vi "图像DCT变换.vi"(11 "图像簇":T1) -> (3 "DCT变换结果":dbl[][][](array[numeric]))   [LabVIEW 2018]
uses:
  <vilib>/Analysis/2dsp.llb/2D DCT.vi
  <vilib>/Analysis/NI_AALPro.lvlib
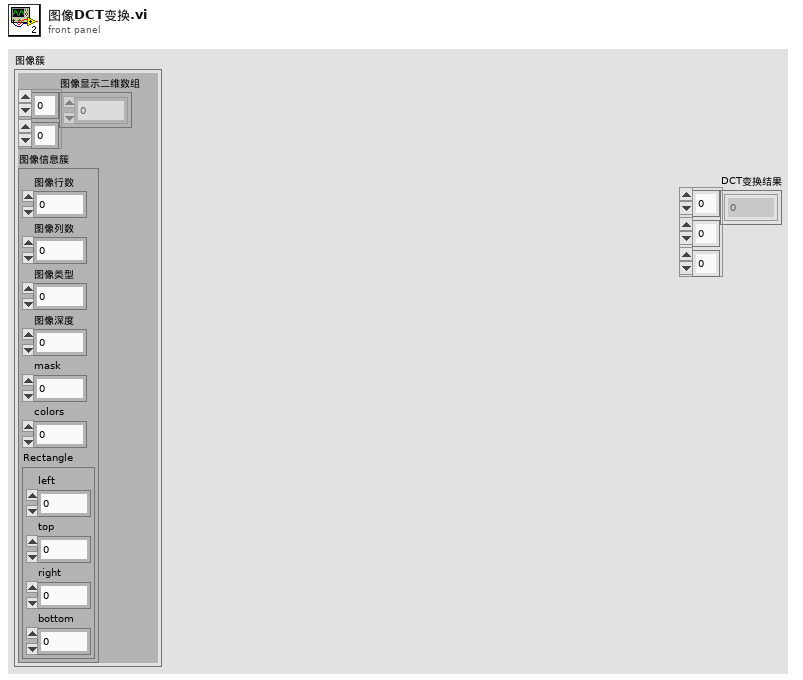
[diagram p1: front panel]
types:
  T1 = cluster{"图像显示二维数组":dbl[][], "图像信息簇":cluster{"图像行数":dbl, "图像列数":dbl, "图像类型":dbl, "图像深度":i32, "mask":i32, "colors":i32, "Rectangle":cluster{"left":i16, "top":i16, "right":i16, "bottom":i16}}}
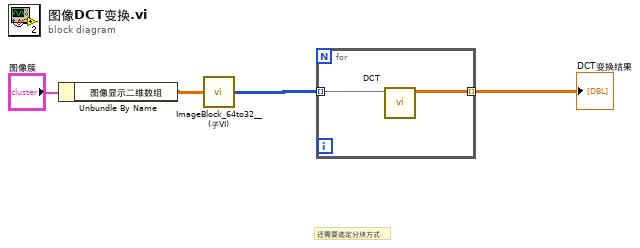
[diagram p0: block diagram]
diagram:
  # "还需要选定分块方式"
  n1 = Unbundle By Name("图像簇") -> ("图像显示二维数组"=w4:dbl[][])
  n2 = call "ImageBlock_64to32__ (子VI).vi"("8-bit pixmap"=w4) -> ("数组"=w3:u8[][][])
  n3 = for {
    tunnel: w3 -> [w6] mode=indexing
    tunnel: [w5] -> w2 mode=indexing
    n4 = call-poly <vilib>:"DCT.vi"("X"=w6) -> ("DCT {X}"=w5:dbl[][])  [unwired: 10 out]
  }
  "DCT变换结果" <- w2
